vi "VI-Replace Event Data.vi"(7 "Create Events method":path, 11 "error in (no error)":errorcluster, 12 "Event Data typedef":path, 13 "Events typedef":path) -> (15 "error out":errorcluster)   [LabVIEW 2015]
uses:
  <vilib>/Utility/traverseref.llb/TRef TravTarget.ctl
  <vilib>/Utility/traverseref.llb/VI Scripting - Traverse.lvlib
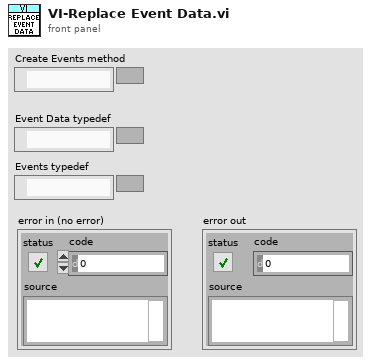
[diagram p1: front panel]
types:
  T1 = typedef "TRef TravTarget.ctl" = enum16{"FP", "BD", "Other"}
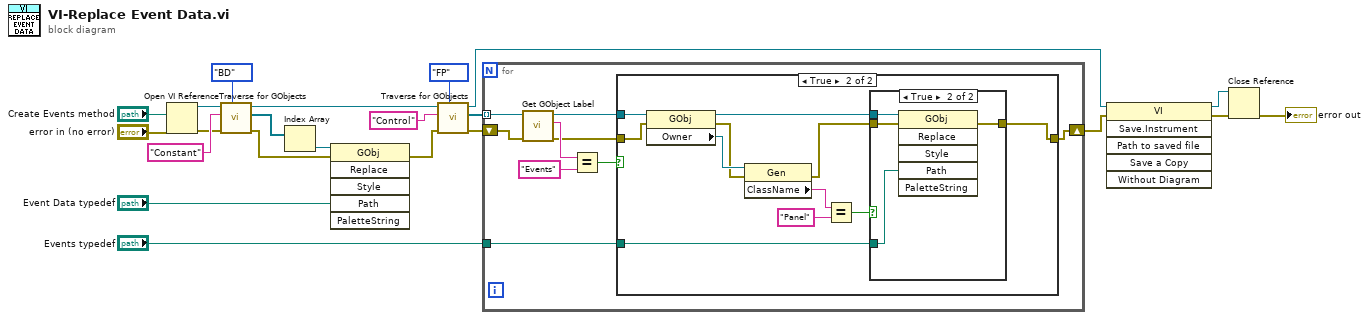
[diagram p0: block diagram]
diagram:
  n1 = Open VI Reference(vi path="Create Events method", error in (no error)="error in (no error)") -> (vi reference=w18:refnum<vi>, error out=w1:errorcluster)  [unwired: 4 in]
  n2 = call <vilib>:"Traverse for GObjects.vi"("Traverse Target"=TRef_TravTarget."BD", "error in (no error)"=w1, "Class Name"="Constant", "VI Refnum"=w18) -> ("error out"=w12:errorcluster, "References"=w14:refnum<vi>[], "dup VI Refnum"=w10:refnum<vi>)  [unwired: 4 in, 1 out]
  n3 = Index Array(array=w14) -> (element=w13:refnum<vi>)  [unwired: 1 in]
  n4 = invoke class="GObj" method="Replace"(reference=w13, error in=w12, "Path"="Event Data typedef") -> (error out=w8:errorcluster)  [unwired: 3 in, 5 out]
  n5 = call <vilib>:"Traverse for GObjects.vi"("Traverse Target"=TRef_TravTarget."FP", "error in (no error)"=w8, "Class Name"="Control", "VI Refnum"=w10) -> ("error out"=w6:errorcluster, "References"=w7:refnum<vi>[], "dup VI Refnum"=w2:refnum<vi>)  [unwired: 4 in, 1 out]
  n6 = for {
    tunnel: w7 -> [w24] mode=indexing
    shift-right: [w27] -> w4
    shift-left: w6 -> [w23]
    tunnel: "Events typedef" -> [w26]
    n7 = call <vilib>:"Get GObject Label.vi"("error in (no error)"=w23, "GObject"=w24) -> ("error out"=w28:errorcluster, "Object Label"=w31:string, "dup GObject"=w29:refnum<vi>)  [unwired: 5 in, 2 out]
    n8 = Equal?(x=w31, y="Events") -> (x = y?=w25:bool)
    n9 = case shown="True" w25 {
      tunnel: w29 -> [_ w38]
      tunnel: w28 -> [w32 w37]
      tunnel: [w32 w43] -> w27
      tunnel: w26 -> [_ w42]
      frame False {
      }
      frame True {
        n10 = property class="GObj"(reference=w38, error in=w37) -> (reference out=w36:refnum<vi>, error out=w40:errorcluster, "Owner"=w41:refnum<vi>)
        n11 = property class="Gen"(reference=w41, error in=w40) -> (error out=w35:errorcluster, "ClassName"=w34:string)  [unwired: 1 out]
        n12 = Equal?(x=w34, y="Panel") -> (x = y?=w33:bool)
        n13 = case shown="True" w33 {
          tunnel: [w44 w48] -> w43
          tunnel: w42 -> [_ w47]
          tunnel: w36 -> [_ w46]
          tunnel: w35 -> [w44 w45]
          frame False {
          }
          frame True {
            n14 = invoke class="GObj" method="Replace"(reference=w46, error in=w45, "Path"=w47) -> (error out=w48:errorcluster)  [unwired: 3 in, 5 out]
          }
        }
      }
    }
  }
  n15 = invoke class="VI" method="Save.Instrument"(reference=w2, error in=w4) -> (reference out=w20:refnum<vi>, error out=w19:errorcluster)  [unwired: 4 in, 4 out]
  n16 = Close Reference(reference=w20, error in (no error)=w19) -> (error out=→"error out":errorcluster)
